vi "Write HDI Slots.vi"(8 "error in (no error)":errorcluster, 10 "HDI Slots":T1(array[cluster]), 11 "WorkTable Class in":refnum<class "WorkTable Class.lvclass">) -> (0 "error out":errorcluster, 3 "WorkTable Class out":refnum<class "WorkTable Class.lvclass">)   [LabVIEW 2011, in "WorkTable Class.lvclass"]
uses:
  WorkTable Class.lvclass
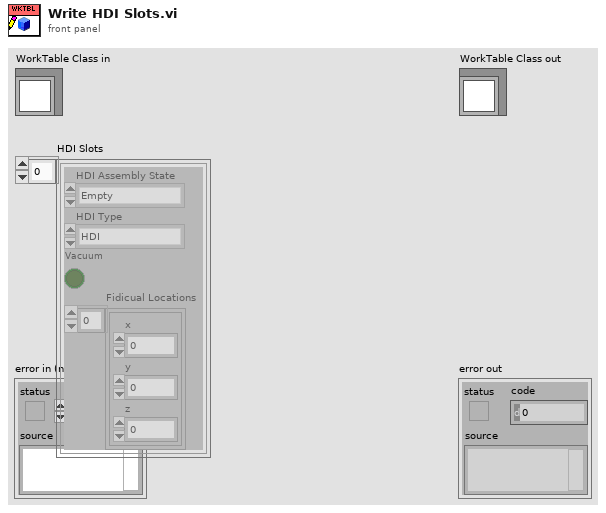
[diagram p1: front panel]
types:
  T1 = cluster{"HDI Assembly State":enum16{"Empty", "Populated"}, "HDI Type":enum16{"HDI", "Polyimide"}, "Vacuum":bool, "Fidicual Locations":cluster{"x":dbl, "y":dbl, "z":dbl}[]}[]
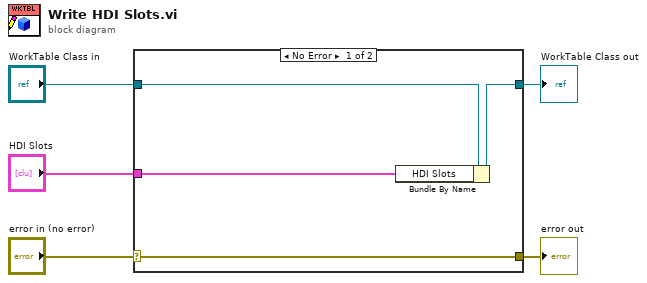
[diagram p0: block diagram]
diagram:
  n1 = case shown="No Error" "error in (no error)" {
    selector: "error in (no error)" -> [w9 w10]
    tunnel: [w9 w10] -> w4
    tunnel: [w7 w11] -> w2
    tunnel: "WorkTable Class in" -> [w8 w11]
    tunnel: "HDI Slots" -> [w6 _]
    frame No Error {
      n2 = Bundle By Name(cluster=w8, "HDI Slots"=w6) -> (w7:refnum<class "WorkTable Class.lvclass">)
    }
    frame Error {
    }
  }
  "error out" <- w4
  "WorkTable Class out" <- w2
